vi "initializer_validate_specs.vi"(9 "Spec File Loaded":bool, 10 "Parameters Tree":refnum<vi>, 11 "# Lines":refnum<vi>) -> (0 "validationErrors":string, 1 "Valid?":bool, 2 "Specifications":string)   [LabVIEW 2019]
uses:
  lib/libSpecValiReader.so
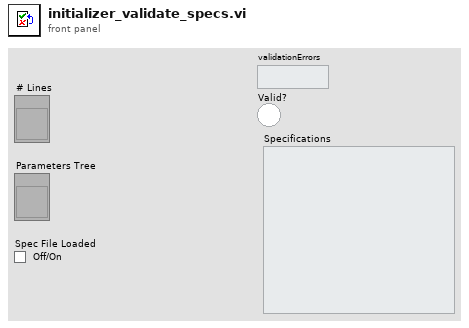
[diagram p1: front panel]
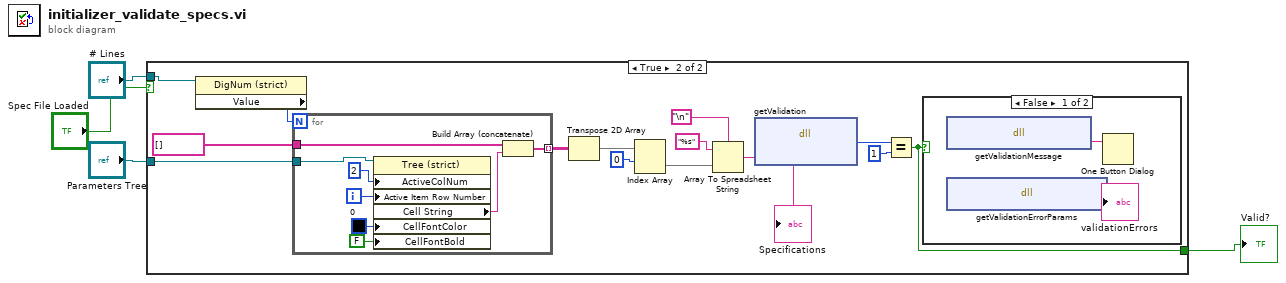
[diagram p0: block diagram]
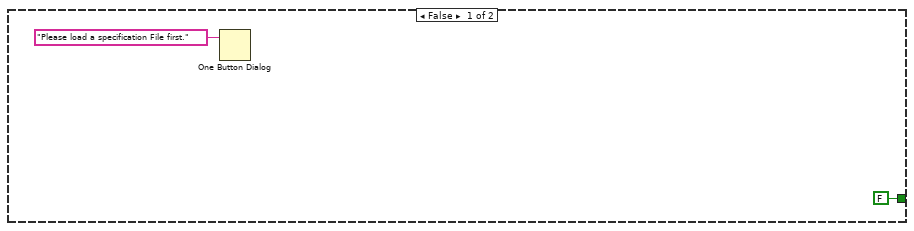
[diagram p2: hidden frame]
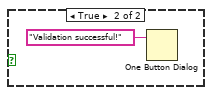
[diagram p3: hidden frame]
diagram:
  n1 = case shown="True" "Spec File Loaded" {
    tunnel: "# Lines" -> [_ w9]
    tunnel: "Parameters Tree" -> [_ w8]
    tunnel: [FALSE w7] -> w1
    frame False {
      n2 = One Button Dialog(message="Please load a specification File first.") -> ()  [unwired: 1 in, 1 out]
    }
    frame True {
      n3 = property class="DigNum (strict)"(reference=w9) -> ("Value"=w20:i32)  [unwired: 1 in, 2 out]
      n4 = for {
        N: w20 -> [_]
        tunnel: string[] [] ("Empty Val Arr") -> [w26]
        tunnel: [w25] -> w18 mode=indexing
        tunnel: w8 -> [w23]
        i -> [w28]
        n5 = property on="Property Node" class="Tree (strict)"(reference=w23, "ActiveColNum"=2 ("Active Cell:Active Column Number"), "Active Item Row Number"=w28, "CellFontColor"=u32 0 ("Active Cell:Cell Font:Color"), "CellFontBold"=FALSE ("Active Cell:Cell Font:Bold")) -> ("Cell String"=w24:string)  [unwired: 1 in, 2 out]
        n6 = Build Array (concatenate)(w26, w24) -> (w25:string[])
      }
      n7 = Transpose 2D Array(2D array=w18) -> (transposed array=w17:string[][])
      n8 = Index Array(array=w17, index (row)=0) -> (element=w16:string[])  [unwired: 1 in]
      n9 = Array To Spreadsheet String(delimiter (Tab)="\n", array=w16, 3:"%s" ("format string")) -> (spreadsheet string=w13:string)
      "Specifications" <- w13
      n10 = dll-call lib="home/paul/Schreibtisch/Biogas_plant_setup/lib/libSpecValiReader.so" fn="getValidation"("inputSpecs"=w13) -> ("isValid"=w12:i32)  [unwired: 4 in, 2 out]
      n11 = Equal?(x=w12, y=1) -> (x = y?=w7:bool)
      n12 = case shown="False" w7 {
        frame False {
          n13 = dll-call lib="home/paul/Schreibtisch/Biogas_plant_setup/lib/libSpecValiReader.so" fn="getValidationMessage"() -> ("validationMessage"=w30:string)  [unwired: 3 in, 2 out]
          n14 = dll-call lib="home/paul/Schreibtisch/Biogas_plant_setup/lib/libSpecValiReader.so" fn="getValidationErrorParams"() -> ("validationErrors"=→"validationErrors":string)  [unwired: 3 in, 2 out]
          n15 = One Button Dialog(message=w30) -> ()  [unwired: 1 in, 1 out]
        }
        frame True {
          n16 = One Button Dialog(message="Validation successful!") -> ()  [unwired: 1 in, 1 out]
        }
      }
    }
  }
  "Valid?" <- w1
